vi "Write stateFactory.vi"(10 "StateFactory.lvlib:StateFactory.lvclass":refnum<class "IStateFactory.lvclass">, 11 "ConcreteContext1 in":refnum<class "ContextThisComponent.lvclass">) -> (3 "ConcreteContext1 out":refnum<class "ContextThisComponent.lvclass">)   [LabVIEW 2012, in "ContextThisComponent.lvclass"]
uses:
  ContextThisComponent.lvclass
  IStateFactory/IStateFactory.lvclass
  ContextThisComponent.lvclass/ContextThisComponent.ctl
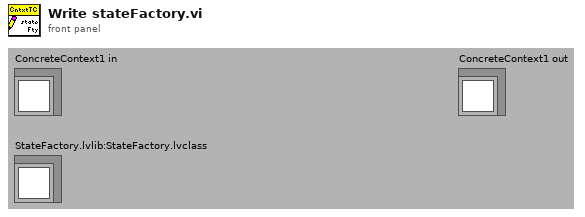
[diagram p1: front panel]
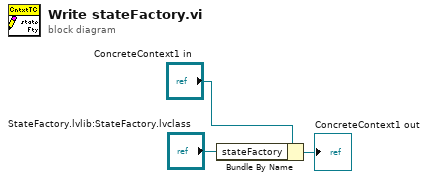
[diagram p0: block diagram]
diagram:
  n1 = Bundle By Name(cluster="ConcreteContext1 in", "stateFactory"="StateFactory.lvlib:StateFactory.lvclass") -> (→"ConcreteContext1 out":refnum<class "ContextThisComponent.lvclass">)
